vi "Map Queue.vi"() -> (3 "Queue out":refnum<queue>)   [LabVIEW 2021, in "d18.lvlib"]
uses:
  d18.lvlib
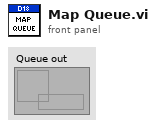
[diagram p1: front panel]
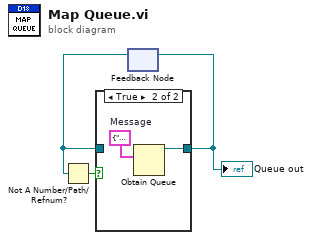
[diagram p0: block diagram]
diagram:
  n1 = feedback #1() -> (w3:refnum<queue>)  [unwired: 1 in]
  n2 = Not A Number/Path/Refnum?(number/path/refnum=w3) -> (NaN/Path/Refnum?=w2:bool)
  n3 = case shown="True" w2 {
    tunnel: [w4 w6] -> w1
    tunnel: w3 -> [w4 _]
    frame False {
    }
    frame True {
      w5 = cluster{"Instruction":string, "Data":variant} {"Instruction"="", "Data"=variant}  # Message
      n4 = Obtain Queue(element data type=w5) -> (queue out=w6:refnum<queue>)  [unwired: 4 in, 2 out]
    }
  }
  "Queue out" <- w1
  n5 = feedback-in #1(w1) -> ()
